vi "Analysis Vol. 3 CSV Read.vi"() -> ()   [LabVIEW 2014] (continued)
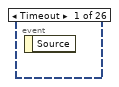
[diagram p2: hidden frame]
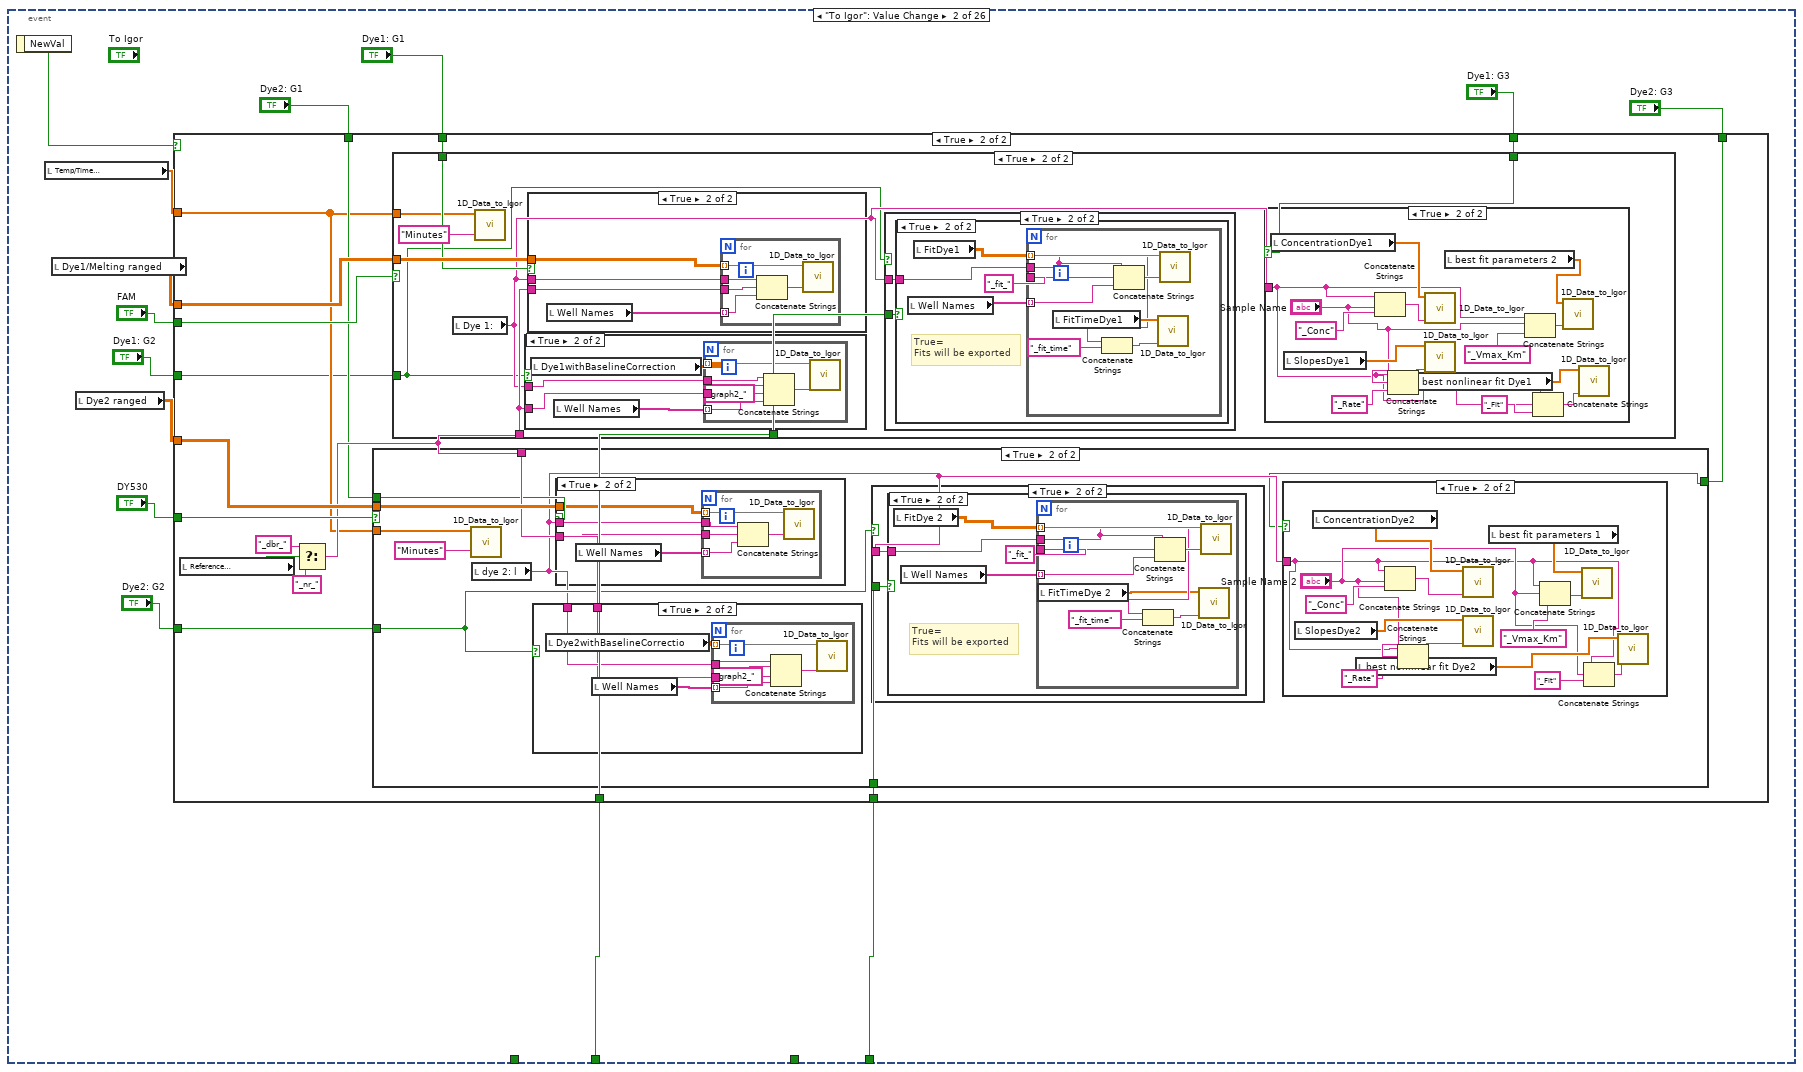
[diagram p3: hidden frame]
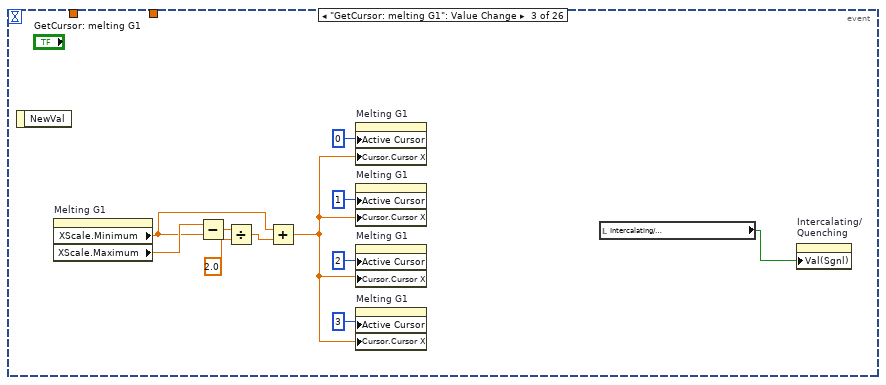
[diagram p17: hidden frame]
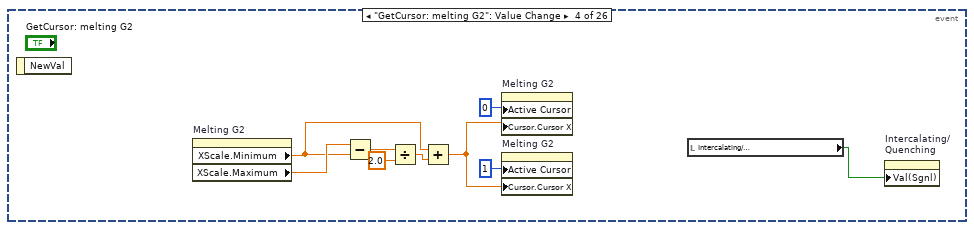
[diagram p18: hidden frame]
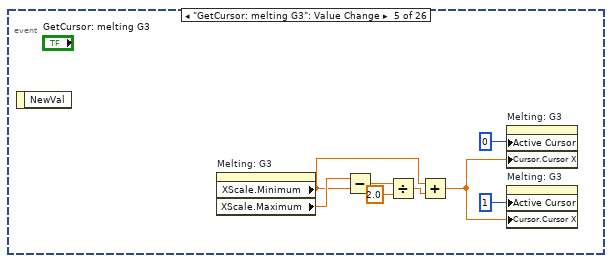
[diagram p19: hidden frame]
              tunnel: w890 -> [w916 w928]
              tunnel: w888 -> [_ w929]
              tunnel: w887 -> [_ w926]
              tunnel: w885 -> [w914 _]
              frame False {
                n546 = for {
                  tunnel: w916 -> [w917] mode=indexing
                  tunnel: w914 -> [w919]
                  tunnel: [w918] -> w915 mode=indexing
                  n547 = case shown="True" w919 {
                    tunnel: w917 -> [w920 w924]
                    tunnel: [w920 w921] -> w918
                    frame False {
                    }
                    frame True {
                      n548 = Array Max & Min(array=w924) -> (max value=w922:dbl)  [unwired: 3 out]
                      n549 = Multiply(x=w924, y=-1.0) -> (x*y=w923:dbl[])
                      n550 = Add(x=w923, y=w922) -> (x+y=w921:dbl[])
                    }
                  }
                }
              }
              frame True {
                n551 = for {
                  tunnel: w929 -> [w939] mode=indexing
                  tunnel: w928 -> [w938] mode=indexing
                  tunnel: [w931] -> w927 mode=indexing
                  tunnel: w926 -> [w930]
                  n552 = Array Max & Min(array=w938) -> (max value=w937:dbl, min value=w936:dbl)  [unwired: 2 out]
                  n553 = Subtract(x=w938, y=w936) -> (x-y=w934:dbl[])
                  n554 = Subtract(x=w937, y=w936) -> (x-y=w933:dbl)
                  n555 = Divide(x=w934, y=w933) -> (x/y=w935:dbl[])
                  n556 = Multiply(x=w935, y=w939) -> (x*y=w932:dbl[])
                  n557 = case shown="False" w930 {
                    tunnel: [w940 w942] -> w931
                    tunnel: w932 -> [w940 w941]
                    frame False {
                    }
                    frame True {
                      n558 = Array Max & Min(array=w941) -> (max value=w943:dbl)  [unwired: 3 out]
                      n559 = Multiply(x=w941, y=-1.0) -> (x*y=w944:dbl[])
                      n560 = Add(x=w944, y=w943) -> (x+y=w942:dbl[])
                    }
                  }
                }
              }
            }
            n561 = case shown="True" w882 {
              tunnel: [w906 w907] -> w883
              tunnel: w884 -> [w906 w908]
              frame False {
              }
              frame True {
                n562 = for {
                  tunnel: w908 -> [w912] mode=indexing
                  tunnel: [w909] -> w907 mode=indexing
                  n563 = Array Max & Min(array=w912) -> (min value=w913:dbl)  [unwired: 3 out]
                  n564 = Subtract(x=w912, y=w913) -> (x-y=w910:dbl[])
                  n565 = Array Max & Min(array=w910) -> (max value=w911:dbl)  [unwired: 3 out]
                  n566 = Divide(x=w910, y=w911) -> (x/y=w909:dbl[])
                }
              }
            }
            "Dye2withBaselineCorrectio" <- w883
            n567 = for {
              tunnel: [w948] -> w886 mode=indexing
              tunnel: w883 -> [w947] mode=indexing
              tunnel: w891 -> [w946]
              # "Create Plots"
              n568 = Bundle("Temp/Time\nranged"=w946, w947) -> (w948:cluster{"Temp/Time\nranged":dbl[], dbl[]})  [unwired: 1 in]
            }
            "Dye 5" <- w886
          }
        }
        n569 = case shown="True" w828 {
          tunnel: w820 -> [w838 _]
          tunnel: w830 -> [w834 _]
          tunnel: w829 -> [_ w858]
          frame True {
            n570 = property on="Dye 5" class="XYGraph (strict)"("Active Cursor"=u32 0, "Active Cursor"=u32 1) -> ("Cursor.Cursor X"=w843:dbl, "Cursor.Cursor X"=w842:dbl)  [unwired: 2 in, 2 out]
            n571 = Max & Min(x=w843, y=w842) -> (max(x,y)=w845:dbl, min(x,y)=w844:dbl)
            n572 = Subtract(x=w845, y=w844) -> (x-y=w841:dbl)
            n573 = Array Subset(array=w834, index (col)=w844, length (col)=w841) -> (w839:dbl[][])  [unwired: 2 in]
            n574 = Array Subset(array=w838, index=w844, length=w841) -> (w840:dbl[])
            n575 = for {
              tunnel: w839 -> [w857] mode=indexing
              tunnel: w840 -> [w849]
              shift-right: [w855] -> w833
              shift-left: cluster{"Y":dbl[], "Y":dbl[]}[] [] ("Dye 3") -> [w854]
              tunnel: w838 -> [w852]
              tunnel: w834 -> [w851] mode=indexing
              tunnel: [w850] -> w836 mode=indexing
              tunnel: [w849] -> w835
              tunnel: [w848] -> w832 mode=indexing
              n576 = call <vilib>:"Linear Fit.vi"("Y"=w857, "X"=w849) -> ("Best Linear Fit"=w850:dbl[], "slope"=w848:dbl)  [unwired: 9 in, 3 out]
              n577 = Bundle("Temp/Time\nranged"=w852, "Dye2 ranged"=w851) -> (w853:T9)  [unwired: 1 in]
              n578 = Bundle(w849, "Best Linear Fit"=w850) -> (w856:cluster{dbl[], "Best Linear Fit":dbl[]})  [unwired: 1 in]
              n579 = Insert Into Array(array=w854, new element #1=w856, new element #2=w853) -> (w855:cluster{"Y":dbl[], "Y":dbl[]}[])  [unwired: 1 in]
            }
            "FitDye 2" <- w836
            "FitTimeDye 2" <- w835
            "FitDye2Slopes" <- w832
            n580 = local write "Dye 5"(w833) -> ()
          }
          frame False {
            n581 = local write "Dye 5"(w858) -> ()
          }
        }
      }
      event "x-axis": Value Change {
        n582 = event-data() -> ("NewVal"=w966:bool)  [unwired: 1 in]
        n583 = Select(t="Temperature [°C]" ("String 2"), s=w966, f="Minutes" ("String")) -> (s? t:f=w965:string)
        n584 = property on="Dye 1: G1" class="XYGraph (strict)"("XScale.NameLbl.Text"=w965) -> ()  [unwired: 2 in, 2 out]
        n585 = property on="Dye 2: G1" class="XYGraph (strict)"("XScale.NameLbl.Text"=w965) -> ()  [unwired: 2 in, 2 out]
        n586 = property on="Dye 4: G2" class="XYGraph (strict)"("XScale.NameLbl.Text"=w965) -> ()  [unwired: 2 in, 2 out]
        n587 = property on="Dye 5: G2" class="XYGraph (strict)"("XScale.NameLbl.Text"=w965) -> ()  [unwired: 2 in, 2 out]
        n588 = property on="REFERENCE G" class="XYGraph (strict)"("XScale.NameLbl.Text"=w965) -> ()  [unwired: 2 in, 2 out]
      }
      event "wells std": Value Change {
        n589 = event-data() -> ()  [unwired: 1 in, 1 out]
        n590 = local write "Well Names"(string[][] [["A1", "A2", "A3", "A4", "A5", "A6", "A7", "A8", "A9", "A10", "A11", "A12"], ["B1", "B2", "B3", "B4", "B5", "B6", "B7", "B8", "B9", "B10", "B11", "B12"], ["C1", "C2", "C3", "C4", "C5", "C6", "C7", "C8", "C9", "C10", "C11", "C12"], ["D1", "D2", "D3", "D4", "D5", "D6", "D7", "D8", "D9", "D10", "D11", "D12"], ["E1", "E2", "E3", "E4", "E5", "E6", "E7", "E8", "E9", "E10", "E11", "E12"], ["F1", "F2", "F3", "F4", "F5", "F6", "F7", "F8", "F9", "F10", "F11", "F12"], ["G1", "G2", "G3", "G4", "G5", "G6", "G7", "G8", "G9", "G10", "G11", "G12"], ["H1", "H2", "H3", "H4", "H5", "H6", "H7", "H8", "H9", "H10", "H11", "H12"]] ("96-well 5")) -> ()
      }
      event "concentration constant": Value Change {
        n591 = event-data() -> ()  [unwired: 1 in, 1 out]
        n592 = local read "Concetrations"() -> (w970:dbl[][])
        n593 = for {
          tunnel: w970 -> [w973] mode=indexing
          tunnel: [w972] -> w971 mode=indexing
          n594 = for {
            tunnel: w973 -> [_] mode=indexing
            tunnel: ["Numeric"] -> w972 mode=indexing
          }
        }
        n595 = local write "Concetrations"(w971) -> ()
      }
      event "concentration horizontal": Value Change {
        n596 = event-data() -> ()  [unwired: 1 in, 1 out]
        n597 = local read "Concetrations"() -> (w976:dbl[][])
        n598 = for {
          tunnel: w976 -> [w984] mode=indexing
          tunnel: w980 -> [w983]
          tunnel: w979 -> [w982]
          tunnel: [w981] -> w975 mode=indexing
          n599 = for {
            tunnel: w984 -> [_] mode=indexing
            tunnel: w983 -> [w989]
            tunnel: w982 -> [w986]
            tunnel: [w987] -> w981 mode=indexing
            i -> [w985]
            n600 = Power Of X(1:w986, 2:w985) -> (0:w988:dbl)
            n601 = Divide(x=w989, y=w988) -> (x/y=w987:dbl)
          }
        }
        n602 = Array Size(array=w976) -> (size(s)=w978:i32[])
        n603 = Index Array(array=w978, index=0) -> ()  [unwired: 1 out]
        n604 = local write "Concetrations"(w975) -> ()
      }
      event "concentration vertical": Value Change {
        n605 = event-data() -> ()  [unwired: 1 in, 1 out]
        n606 = local read "Concetrations"() -> (w993:dbl[][])
        n607 = Transpose 2D Array(2D array=w993) -> (transposed array=w992:dbl[][])
        n608 = for {
          tunnel: w992 -> [w1001] mode=indexing
          tunnel: w997 -> [w1000]
          tunnel: w996 -> [w999]
          tunnel: [w998] -> w991 mode=indexing
          n609 = for {
            tunnel: w1001 -> [_] mode=indexing
            tunnel: w1000 -> [w1006]
            tunnel: w999 -> [w1003]
            tunnel: [w1004] -> w998 mode=indexing
            i -> [w1002]
            n610 = Power Of X(1:w1003, 2:w1002) -> (0:w1005:dbl)
            n611 = Divide(x=w1006, y=w1005) -> (x/y=w1004:dbl)
          }
        }
        n612 = Array Size(array=w992) -> (size(s)=w995:i32[])
        n613 = Index Array(array=w995, index=0) -> ()  [unwired: 1 out]
        n614 = Transpose 2D Array(2D array=w991) -> (transposed array=w990:dbl[][])
        n615 = local write "Concetrations"(w990) -> ()
      }
      event "Reference \non/off", "Choose Range:": Value Change {
        # "CREATE PLOTS"
        # "DIVIDE BY REFERENCE"
        n616 = event-data() -> ()  [unwired: 1 in, 1 out]
        n617 = local read "Choose Range:"() -> (w1009:cluster{dbl, dbl})
        n618 = local read "Dye 1/Melting"() -> (w1018:dbl[][])
        n619 = local read "Temp/Time"() -> (w1021:dbl[])
        n620 = local read "reference"() -> (w1020:dbl[][])
        n621 = local read "Dye 2"() -> (w1019:dbl[][])
        n622 = Unbundle(w1009) -> (w1026:dbl, w1025:dbl)
        n623 = Max & Min(x=w1026, y=w1025) -> (max(x,y)=w1023:dbl, min(x,y)=w1024:dbl)
        n624 = case shown="True" "On/off" {
          tunnel: [w1030 w1038] -> w1007
          tunnel: w1021 -> [w1030 w1035]
          tunnel: [w1029 w1042] -> w1014
          tunnel: w1018 -> [w1029 w1047]
          tunnel: [w1028 w1041] -> w1015
          tunnel: w1019 -> [w1028 w1046]
          tunnel: w1020 -> [w1027 w1040]
          tunnel: [w1027 w1039] -> w1017
          frame False {
          }
          frame True {
            n625 = Unbundle("Choose Range:") -> (w1044:dbl, w1045:dbl)
            n626 = Max & Min(x=w1044, y=w1045) -> (max(x,y)=w1036:dbl, min(x,y)=w1037:dbl)
            n627 = Threshold 1D Array(2:w1037, 3:w1035) -> (0:w1033:dbl)  [unwired: 1 in]
            n628 = Threshold 1D Array(2:w1036, 3:w1035) -> (0:w1034:dbl)  [unwired: 1 in]
            n629 = Round Toward +Infinity(x=w1034) -> (ceil(x): smallest int >= x=w1031:dbl)
            n630 = Round Toward -Infinity(1:w1033) -> (0:w1032:dbl)
            n631 = for {
              tunnel: w1035 -> [w1058]
              tunnel: w1047 -> [w1057] mode=indexing
              tunnel: w1046 -> [w1056] mode=indexing
              tunnel: [w1055] -> w1042 mode=indexing
              tunnel: [w1053] -> w1041 mode=indexing
              tunnel: [w1054] -> w1038
              tunnel: w1040 -> [w1051] mode=indexing
              tunnel: [w1050] -> w1039 mode=indexing
              tunnel: w1031 -> [w1049]
              tunnel: w1032 -> [w1048]
              n632 = Subtract(x=w1049, y=w1048) -> (x-y=w1052:dbl)
              n633 = Array Subset(array=w1058, index=w1048, length=w1052) -> (w1054:dbl[])
              n634 = Array Subset(array=w1057, index=w1048, length=w1052) -> (w1055:dbl[])
              n635 = Array Subset(array=w1056, index=w1048, length=w1052) -> (w1053:dbl[])
              n636 = Array Subset(array=w1051, index=w1048, length=w1052) -> (w1050:dbl[])
            }
          }
        }
        "Temp/Time\nranged" <- w1007
        n637 = Subtract(x=w1023, y=w1024) -> (x-y=w1022:dbl)
        n638 = disable-structure shown="Disabled" {
          disable-tunnel: w1022 -> [w1071 _]
          frame Disabled {
            w1072 = 3.0 ("y")
            w1089 = u32 1 ("Active Cursor")
            w1088 = u32 0 ("Active Cursor")
            w1090 = u32 1 ("Active Cursor")
            w1091 = u32 0 ("Active Cursor")
            w1092 = 3.0 ("y")
            w1109 = u32 1 ("Active Cursor")
            w1108 = u32 0 ("Active Cursor")
            w1110 = u32 1 ("Active Cursor")
            w1111 = u32 0 ("Active Cursor")
            n639 = property on="Dye 2: G1" class="XYGraph (strict)"("Active Cursor"=w1111, "Active Cursor"=w1110) -> ("Cursor.Cursor X"=w1096:dbl, "Cursor.Cursor X"=w1097:dbl)  [unwired: 2 in, 2 out]
            n640 = property on="Dye 1: G1" class="XYGraph (strict)"("Active Cursor"=w1111, "Active Cursor"=w1110) -> ("Cursor.Cursor X"=w1098:dbl, "Cursor.Cursor X"=w1099:dbl)  [unwired: 2 in, 2 out]
            n641 = Greater?(x=w1097, y=w1071) -> (0:w1103:bool)
            n642 = Greater?(x=w1096, y=w1071) -> (0:w1102:bool)
            n643 = Greater?(x=w1098, y=w1071) -> (0:w1101:bool)
            n644 = Greater?(x=w1099, y=w1071) -> (0:w1107:bool)
            n645 = Subtract(x=w1071, y=w1092) -> (x-y=w1100:dbl)
            n646 = Add(x=w1092, y=w1100) -> (x+y=w1094:dbl)
            n647 = Add(x=w1092, y=w1100) -> (x+y=w1093:dbl)
            n648 = Select(t=w1100, s=w1103, f=w1097) -> (s? t:f=w1104:dbl)
            n649 = Select(t=w1094, s=w1102, f=w1096) -> (s? t:f=w1105:dbl)
            n650 = Select(t=w1093, s=w1101, f=w1098) -> (s? t:f=w1095:dbl)
            n651 = Select(t=w1100, s=w1107, f=w1099) -> (s? t:f=w1106:dbl)
            n652 = property on="Dye 2: G1" class="XYGraph (strict)"("Active Cursor"=w1108, "Cursor.Cursor X"=w1105, "Active Cursor"=w1109, "Cursor.Cursor X"=w1104) -> ()  [unwired: 2 in, 2 out]
            n653 = property on="Dye 1: G1" class="XYGraph (strict)"("Active Cursor"=w1108, "Cursor.Cursor X"=w1095, "Active Cursor"=w1109, "Cursor.Cursor X"=w1106) -> ()  [unwired: 2 in, 2 out]
            n654 = property on="Dye 1: G2" class="XYGraph (strict)"("Active Cursor"=w1091, "Active Cursor"=w1090) -> ("Cursor.Cursor X"=w1076:dbl, "Cursor.Cursor X"=w1077:dbl)  [unwired: 2 in, 2 out]
            n655 = property on="Dye 2: G2" class="XYGraph (strict)"("Active Cursor"=w1091, "Active Cursor"=w1090) -> ("Cursor.Cursor X"=w1078:dbl, "Cursor.Cursor X"=w1079:dbl)  [unwired: 2 in, 2 out]
            n656 = Greater?(x=w1076, y=w1071) -> (0:w1082:bool)
            n657 = Greater?(x=w1077, y=w1071) -> (0:w1083:bool)
            n658 = Greater?(x=w1078, y=w1071) -> (0:w1081:bool)
            n659 = Greater?(x=w1079, y=w1071) -> (0:w1087:bool)
            n660 = Subtract(x=w1071, y=w1072) -> (x-y=w1080:dbl)
            n661 = Add(x=w1072, y=w1080) -> (x+y=w1074:dbl)
            n662 = Add(x=w1072, y=w1080) -> (x+y=w1073:dbl)
            n663 = Select(t=w1074, s=w1082, f=w1076) -> (s? t:f=w1085:dbl)
            n664 = Select(t=w1080, s=w1083, f=w1077) -> (s? t:f=w1084:dbl)
            n665 = Select(t=w1073, s=w1081, f=w1078) -> (s? t:f=w1075:dbl)
            n666 = Select(t=w1080, s=w1087, f=w1079) -> (s? t:f=w1086:dbl)
            n667 = property on="Dye 1: G2" class="XYGraph (strict)"("Active Cursor"=w1088, "Cursor.Cursor X"=w1085, "Active Cursor"=w1089, "Cursor.Cursor X"=w1084) -> ()  [unwired: 2 in, 2 out]
            n668 = property on="Dye 2: G2" class="XYGraph (strict)"("Active Cursor"=w1088, "Cursor.Cursor X"=w1075, "Active Cursor"=w1089, "Cursor.Cursor X"=w1086) -> ()  [unwired: 2 in, 2 out]
          }
          frame Enabled {
          }
        }
        n669 = case shown="False" "Reference \non/off" {
          tunnel: w1014 -> [w1064 w1066]
          tunnel: w1017 -> [_ w1068]
          tunnel: [w1064 w1070] -> w1012
          tunnel: w1015 -> [w1065 w1069]
          tunnel: [w1065 w1067] -> w1013
          frame False {
          }
          frame True {
            n670 = Divide(x=w1066, y=w1068) -> (x/y=w1070:dbl[][])
            n671 = Divide(x=w1069, y=w1068) -> (x/y=w1067:dbl[][])
          }
        }
        "Dye1/Melting ranged" <- w1012
        "Dye2 ranged" <- w1013
        n672 = for {
          tunnel: w1013 -> [w1063] mode=indexing
          tunnel: [w1061] -> w1008 mode=indexing
          tunnel: [w1062] -> w1010 mode=indexing
          tunnel: w1007 -> [w1059]
          tunnel: w1012 -> [w1060] mode=indexing
          n673 = Bundle("Temp/Time"=w1059, "Dye 1/Melting"=w1060) -> (w1062:T10)  [unwired: 1 in]
          n674 = Bundle("Temp/Time"=w1059, "Dye 2"=w1063) -> (w1061:cluster{"Temp/Time":dbl[], "Dye 2":dbl[]})  [unwired: 1 in]
        }
        n675 = local write "Dye 1: G1"(w1010) -> ()
        n676 = local write "Dye 2: G1"(w1008) -> ()
        n677 = local write "Melting G1"(w1008) -> ()
      }
    }
    "dye 1: k" <- "Dye 1:"
    "dye 1: i" <- "Dye 1:"
    "dye 2: k" <- "dye 2: l"
    "dye 2: i" <- "dye 2: l"
  }
